vi "write_dwelltime_command.vi"(11 "Dwell Time (s)":dbl) -> (3 "Command Out":string)   [LabVIEW 2015]
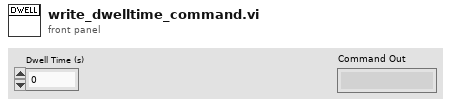
[diagram p1: front panel]
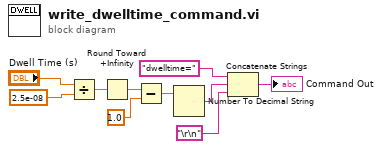
[diagram p0: block diagram]
diagram:
  n1 = Divide(x="Dwell Time (s)", y=2.5e-08) -> (x/y=w8:dbl)
  n2 = Round Toward +Infinity(x=w8) -> (ceil(x): smallest int >= x=w7:dbl)
  n3 = Subtract(x=w7, y=1.0) -> (x-y=w4:dbl)
  n4 = Number To Decimal String(number=w4) -> (decimal integer string=w3:string)  [unwired: 1 in]
  n5 = Concatenate Strings("dwelltime=" ("string"), w3, "\r\n") -> (→"Command Out":string)
